vi "Save to PDF File using BullZip 2009.vi"(8 "error in":errorcluster, 9 "PDF Settings":T1={"ShowPDF"="no", "ShowSettings"="never", "ShowSaveAS"="never", "ShowProgress"="no", "ShowProgressFinished"="no", "ConfirmOverwrite"="no", "RememberLastFileName"="no", "RememberLastFolderName"="no", "WaterMarkText"="", "Author"="", "Title"="", "Subject"=""}, 10 "Save PDF File Path":path) -> (0 "error out":errorcluster caption="Fehler (Ausgang)")   [LabVIEW 2020, in "Linearisierung v2.lvlib" / "Protokoll.lvlib"]
uses:
  Protokoll.lvlib
  Bullzip.PdfWriter
panel:
  # "Save to PDF File using BullZip PDF Printer"
  # "Download Freeware BullZip PDF Printer and install.\nBullZip Reference:\n\nhttp://www.bullzip.com/products/pdf/info.php"
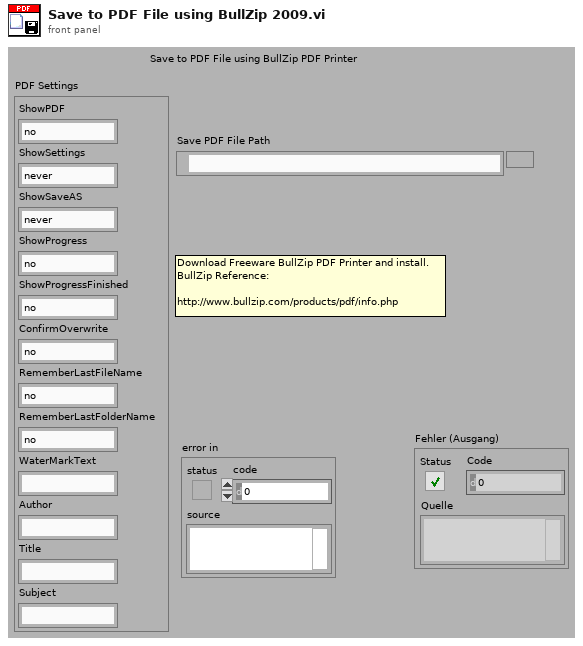
[diagram p1: front panel]
types:
  T1 = cluster{"ShowPDF":string, "ShowSettings":string, "ShowSaveAS":string, "ShowProgress":string, "ShowProgressFinished":string, "ConfirmOverwrite":string, "RememberLastFileName":string, "RememberLastFolderName":string, "WaterMarkText":string, "Author":string, "Title":string, "Subject":string}
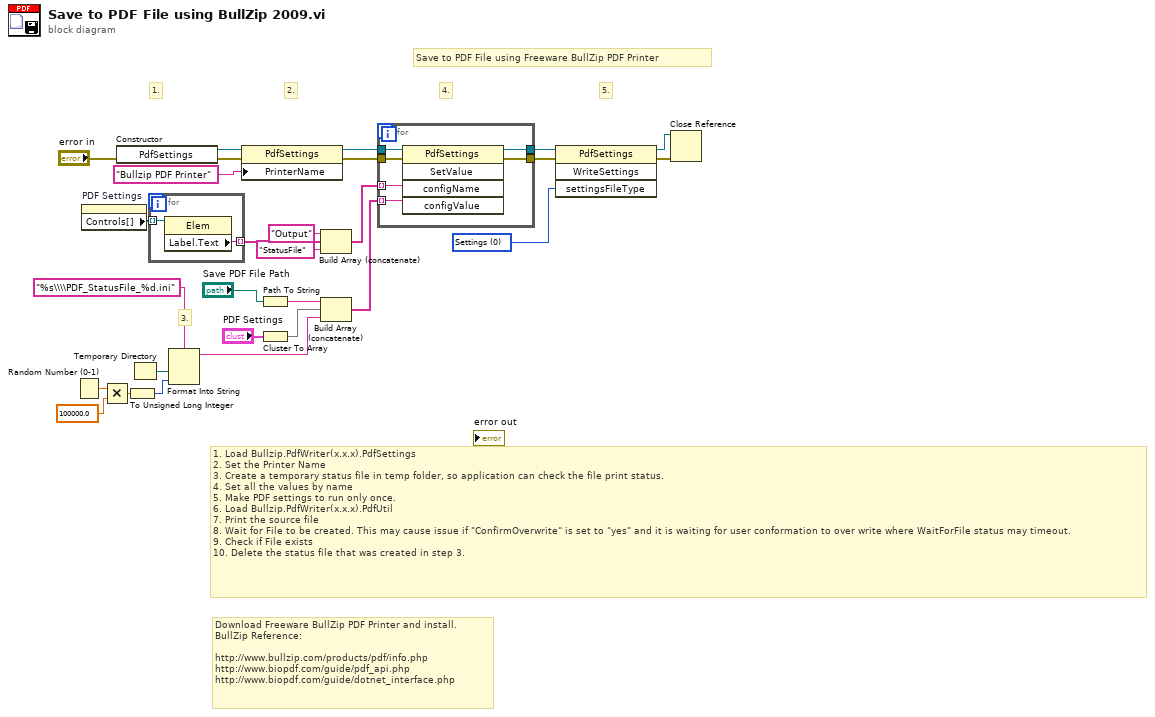
[diagram p0: block diagram]
diagram:
  w11 = 0 items=["Settings", "User", "RunOnce", "Global", "Defaults"] ("settingsFileType")
  # "3."
  # "5."
  # "4."
  # "2."
  # "1."
  # "1.\tLoad Bullzip.PdfWriter(x.x.x).PdfSettings \n2.\tSet the Printer Name\n3.\tCreate a temporary status file in temp folder, so application can check the file print status.\n4.\tSet all the values by name\n5.\tMake PDF settings to run only once.\n6.\tLoad Bullzip.PdfWriter(x.x.x).PdfUtil\n7.\tPrint the source file \n8.\tWait for File to be created. This may cause issue if \"ConfirmOverwrite\" is set to \"yes\" and it is waiting for user conformation to over write where WaitForFile status may timeout.\n9.\tCheck if File exists\n10.\tDelete the status file that was created in step 3."
  # "Save to PDF File using Freeware BullZip PDF Printer"
  # "Download Freeware BullZip PDF Printer and install.\nBullZip Reference:\n\nhttp://www.bullzip.com/products/pdf/info.php\nhttp://www.biopdf.com/guide/pdf_api.php\nhttp://www.biopdf.com/guide/dotnet_interface.php"
  n1 = Random Number (0-1)() -> (number: 0 to 1=w5:dbl)
  n2 = property on="PDF Settings" class="Cluster (strikt)"() -> ("Controls[]"=w20:refnum<vi>[])  [unwired: 2 in, 2 out]
  n3 = Multiply(x=w5, y=100000.0) -> (x*y=w3:dbl)
  n4 = constructor class="PdfSettings" ("Constructor Node")(error in="error in") -> (reference out=w16:refnum<k24>, error out=w28:errorcluster)  [unwired: 2 in, 1 out]
  n5 = To Unsigned Long Integer(number=w3) -> (unsigned 32bit integer=w2:u32)
  n6 = Temporary Directory() -> (w6:path)
  n7 = for {
    tunnel: w20 -> [w30] mode=indexing
    tunnel: [w29] -> w18 mode=indexing
    n8 = property class="Elem"(reference=w30) -> ("Label.Text"=w29:string)  [unwired: 1 in, 2 out]
  }
  n9 = Format Into String(format string="%s\\\\PDF_StatusFile_%d.ini", w6, w2) -> (resulting string=w14:string)  [unwired: 2 in, 1 out]
  n10 = property class="PdfSettings"(reference=w16, error in=w28, "PrinterName"="Bullzip PDF Printer") -> (reference out=w12:refnum<k24>, error out=w27:errorcluster)
  n11 = Path To String(path="Save PDF File Path") -> (string=w24:string)
  n12 = Cluster To Array(cluster="PDF Settings") -> (array=w21:string[])
  n13 = Build Array (concatenate)("Output", w18, "StatusFile") -> (w17:string[])
  n14 = Build Array (concatenate)(w24, w21, w14) -> (w23:string[])
  n15 = for {
    tunnel: w12 -> [w36]
    tunnel: w17 -> [w34] mode=indexing
    tunnel: w23 -> [w33] mode=indexing
    tunnel: [w35] -> w7
    tunnel: w27 -> [w32]
    tunnel: [w31] -> w10
    n16 = invoke class="PdfSettings" method="SetValue"(reference=w36, error in=w32, "configName"=w34, "configValue"=w33) -> (reference out=w35:refnum<k24>, error out=w31:errorcluster)  [unwired: 1 in, 3 out]
  }
  n17 = invoke class="PdfSettings" method="WriteSettings"(reference=w7, error in=w10, "settingsFileType"=w11) -> (reference out=w8:refnum<k24>, error out=w9:errorcluster)  [unwired: 1 in, 2 out]
  n18 = Close Reference(reference=w8, error in (no error)=w9) -> ()  [unwired: 1 out]
